vi "working_gyro.vi"(10 "Parâmetros Iniciais":T1={"Gyro Port"=0, "Sensor - Left"=3, "Sensor - Right"=2, "     Color \nSensor Port"=1, "Kp Front"=0.5, "Motor speed"=-15, "Distance to street"=15.0, "Motor speed turns"=16, "Kp Curvas"=0.3} {"Kp Front" format="%.3f"; "Color \nSensor Port" items=["Port 1", "Port 2", "Port 3", "Port 4"]; "Sensor - Right" items=["Port 1", "Port 2", "Port 3", "Port 4"]; "Sensor - Left" items=["Port 1", "Port 2", "Port 3", "Port 4"]; "Gyro Port" items=["Port 1", "Port 2", "Port 3", "Port 4"]}, 11 "NXT/EV3":T3) -> (0 "NXT/EV3 2":T3)   [LabVIEW 2016]
uses:
  <vilib>/NXT/Subs/LVHSConnector.ctl
  <vilib>/NXT/LegoClasses/BrickReference/BrickReference.lvclass
  parametros.ctl
  <vilib>/NXT/Block Support/NXT_InputPort.ctl
  <vilib>/NXT/Block Support/NXT_OutputPort.ctl
  <vilib>/NXT/Dual Mode Library/Display/clearDisplay.vi
  <vilib>/NXT/NXTIO Xnodes/NXTIONodeSubVIs/NXTStopMotors.vi
  <vilib>/NXT/Dual Mode Library/Display/drawText_Center.vi
  <vilib>/NXT/Dual Mode Library/Sensors/EV3_Gyro_Reset.vi
  <vilib>/NXT/Dual Mode Library/Sensors/EV3_Gyro_Rate.vi
  <vilib>/NXT/Dual Mode Library/Sensors/EV3_Gyro_Angle.vi
  <vilib>/NXT/NXTIO Xnodes/AddressXNode/NXTIOAddress.xnode
  <vilib>/NXT/NXTIO Xnodes/NXTIOXNode/NXTIO.xnode
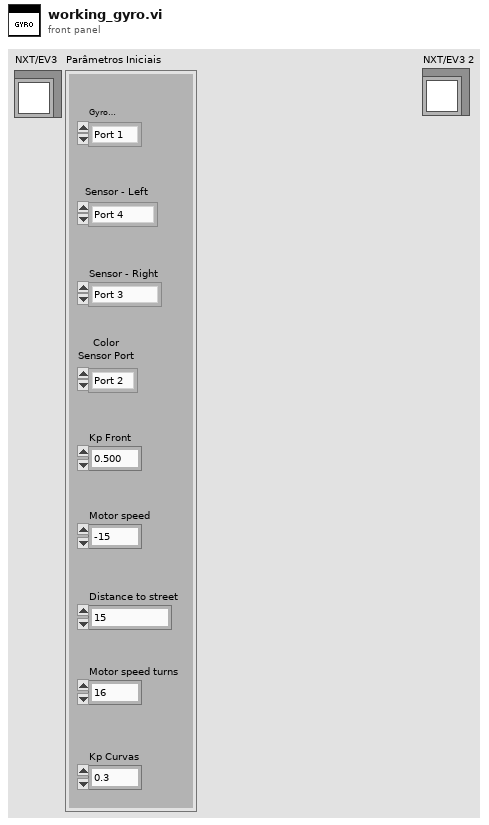
[diagram p1: front panel]
types:
  T1 = typedef "parametros.ctl" = cluster{"Gyro Port":T2, "Sensor - Left":T2, "Sensor - Right":T2, "     Color \nSensor Port":T2, "Kp Front":dbl, "Motor speed":i32, "Distance to street":dbl, "Motor speed turns":i32, "Kp Curvas":dbl}
  T2 = typedef "NXT_InputPort.ctl" = u32
  T3 = typedef "LVHSConnector.ctl" = refnum<class "BrickReference.lvclass">
  T4 = typedef "NXT_OutputPort.ctl" = u8
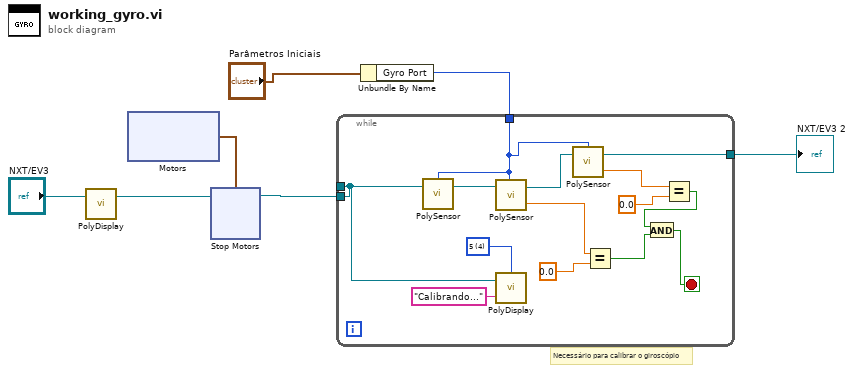
[diagram p0: block diagram]
diagram:
  # "Necessário para calibrar o giroscópio"
  n1 = call-poly <vilib>:"PolyDisplay.vi"("NXT/EV3"="NXT/EV3") -> ("NXT/EV3"=w2:T3)  [unwired: 3 in]
  n2 = xnode "Motors"() -> ("Motor"=w3:cluster{"Port":T4, "Port":T4})
  n3 = xnode "Stop Motors"("Motors"=w3, "NXT/EV3"=w2) -> ("NXT/EV3"=w1:T3)
  n4 = Unbundle By Name("Parâmetros Iniciais") -> ("Gyro Port"=w4:T2)
  n5 = while {
    tunnel: w4 -> [w9]
    tunnel: [w8] -> _
    tunnel: [w12] -> w6
    tunnel: w1 -> [w8]
    stop <- w14 stop-if-true
    w10 = i16 4 items=["1", "2", "3", "4", "5", "6", "7", "8", "9", "10", "11", "12"] ("Line")
    n6 = call-poly <vilib>:"PolySensor.vi"("NXT/EV3"=w8, "Port (Port 1)"=w9) -> ("NXT/EV3"=w20:T3)  [unwired: 2 in]
    n7 = call-poly <vilib>:"PolySensor.vi"("NXT/EV3"=w20, "Port (Port 1)"=w9) -> ("Degrees/Second"=w19:sgl, "NXT/EV3"=w13:T3)  [unwired: 1 in]
    n8 = call-poly <vilib>:"PolyDisplay.vi"("Text"="Calibrando...", "NXT/EV3"=w8, "Line"=w10) -> ()  [unwired: 1 in, 1 out]
    n9 = call-poly <vilib>:"PolySensor.vi"("NXT/EV3"=w13, "Port (Port 1)"=w9) -> ("Degrees"=w16:sgl, "NXT/EV3"=w12:T3)  [unwired: 1 in]
    n10 = Equal?(x=w19, y=sgl 0.0) -> (x = y?=w18:bool)
    n11 = Equal?(x=w16, y=sgl 0.0) -> (x = y?=w15:bool)
    n12 = And(x=w15, y=w18) -> (x .and. y?=w14:bool)
  }
  "NXT/EV3 2" <- w6
